vi "Limelight.vi"() -> (1 "RightTargetNorm":T1, 3 "LeftTargetNorm":T1)   [LabVIEW 2018]
uses:
  Util/Math/Vector/Vector3D.ctl
  5bda4818-5db7-4a37-94fe-e126cb2a47b4.vi
  65baa005-36a5-4b5c-ad00-e7831b38fc40.vi
  ffe1e7bf-722c-4abf-afb3-08bbb05ce56e.vi
  cfa8c977-f46c-4ebb-8e7e-f5b631340d2e.vi
  20f04a56-a653-4d81-a16d-e2cce2d6ced9.vi
  75f726a3-edf9-46da-8158-0b1851abcaf1.vi
  6606baff-e82b-4fed-8c44-0260f9793549.vi
  <vilib>/Array/Sort 2D Array - Pop Stack.vi
  <vilib>/Array/Sort 2D Array - Push Stack.vi
  <vilib>/Rock Robotics/Network Tables/NT Read Numeric Array.vi
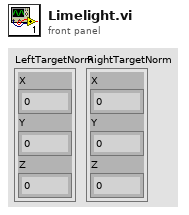
[diagram p1: front panel]
types:
  T1 = typedef "Vector3D.ctl" = cluster{"X":dbl, "Y":dbl, "Z":dbl}
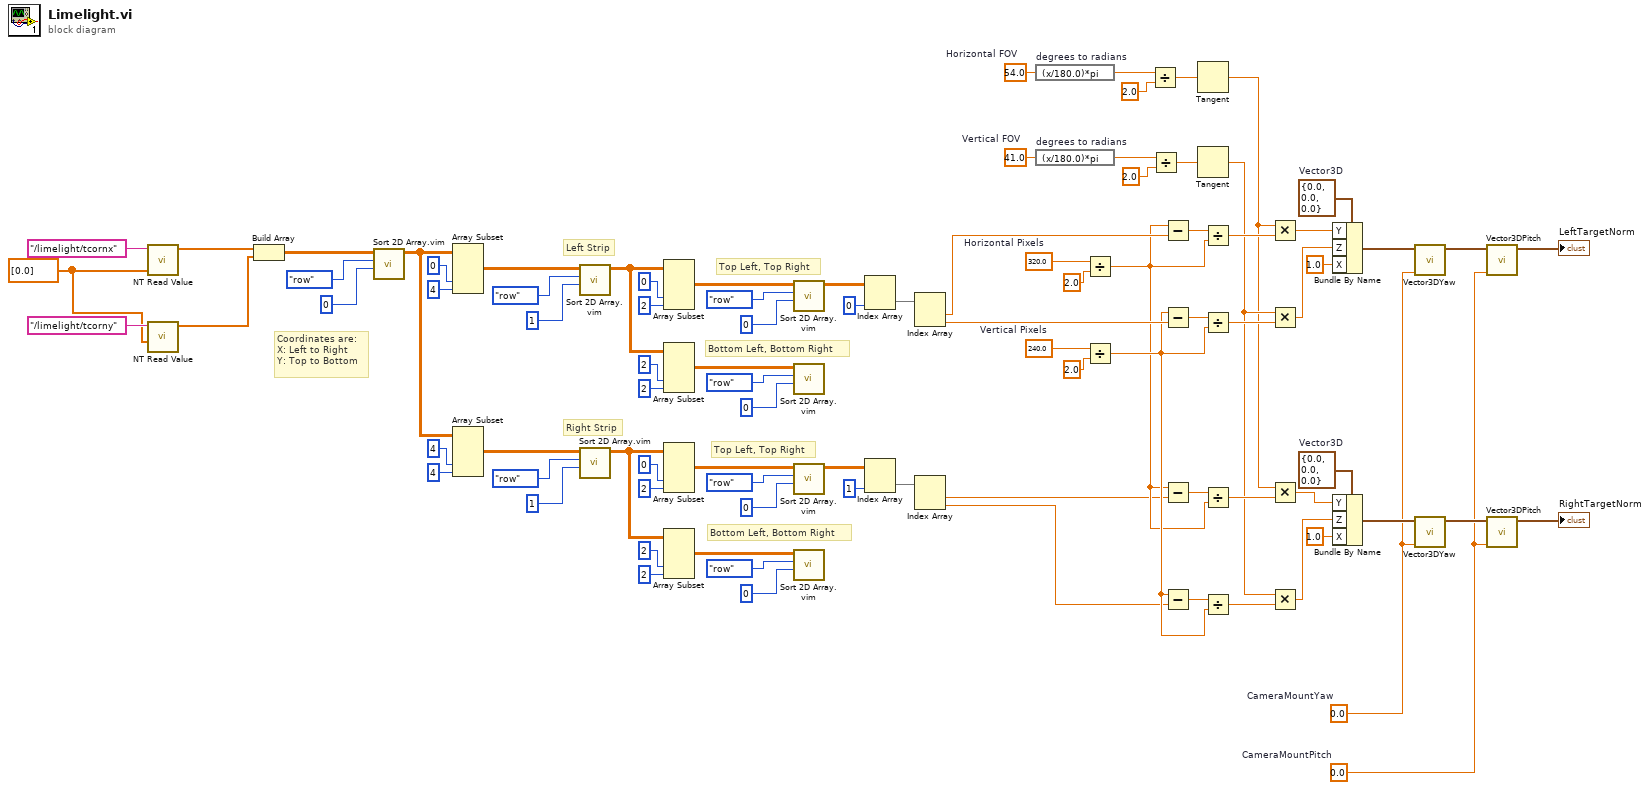
[diagram p0: block diagram]
diagram:
  w2 = 0.0  # CameraMountPitch
  w1 = 0.0  # CameraMountYaw
  w19 = T1 {"X"=0.0, "Y"=0.0, "Z"=0.0}  # Vector3D
  w32 = 320.0  # Horizontal Pixels
  w24 = T1 {"X"=0.0, "Y"=0.0, "Z"=0.0}  # Vector3D
  w38 = 240.0  # Vertical Pixels
  w41 = 54.0  # Horizontal FOV
  w44 = 41.0  # Vertical FOV
  w87 = dbl[] [0.0] ("Default Value")
  # "Coordinates are:\nX: Left to Right\nY: Top to Bottom"
  # "Top Left, Top Right"
  # "Bottom Left, Bottom Right"
  # "Top Left, Top Right"
  # "Bottom Left, Bottom Right"
  # "Right Strip"
  # "Left Strip"
  n1 = call-poly <vilib>:"NT Read Value.vi"("Default Value"=w87, "Name"="/limelight/tcornx") -> ("Numeric Array"=w89:dbl[])  [unwired: 8 in, 1 out]
  n2 = call-poly <vilib>:"NT Read Value.vi"("Default Value"=w87, "Name"="/limelight/tcorny") -> ("Numeric Array"=w88:dbl[])  [unwired: 8 in, 1 out]
  n3 = Build Array(w89, w88) -> (w84:dbl[][])
  n4 = call "Sort 2D Array.vim"("index"=0, "dimension to index (column)"=enum16{"column", "row"}."row", "2D array"=w84) -> ("sorted 2D array"=w79:dbl[][])  [unwired: 7 in, 1 out]
  n5 = Array Subset(array=w79, index (col)=0 ("index"), length (col)=4 ("index")) -> (w76:dbl[][])  [unwired: 2 in]
  n6 = Array Subset(array=w79, index (col)=4 ("index"), length (col)=4 ("index")) -> (w73:dbl[][])  [unwired: 2 in]
  n7 = call "Sort 2D Array.vim"("index"=1, "dimension to index (column)"=enum16{"column", "row"}."row", "2D array"=w76) -> ("sorted 2D array"=w68:dbl[][])  [unwired: 7 in, 1 out]
  n8 = call "Sort 2D Array.vim"("index"=1, "dimension to index (column)"=enum16{"column", "row"}."row", "2D array"=w73) -> ("sorted 2D array"=w63:dbl[][])  [unwired: 7 in, 1 out]
  n9 = Array Subset(array=w68, index (col)=0 ("index"), length (col)=2 ("index")) -> (w60:dbl[][])  [unwired: 2 in]
  n10 = Array Subset(array=w68, index (col)=2 ("index"), length (col)=2 ("index")) -> (w57:dbl[][])  [unwired: 2 in]
  n11 = Array Subset(array=w63, index (col)=0 ("index"), length (col)=2 ("index")) -> (w52:dbl[][])  [unwired: 2 in]
  n12 = Array Subset(array=w63, index (col)=2 ("index"), length (col)=2 ("index")) -> (w51:dbl[][])  [unwired: 2 in]
  n13 = call "Sort 2D Array.vim"("index"=0, "dimension to index (column)"=enum16{"column", "row"}."row", "2D array"=w60) -> ("sorted 2D array"=w48:dbl[][])  [unwired: 7 in, 1 out]
  n14 = call "Sort 2D Array.vim"("index"=0, "dimension to index (column)"=enum16{"column", "row"}."row", "2D array"=w57) -> ()  [unwired: 7 in, 2 out]
  n15 = call "Sort 2D Array.vim"("index"=0, "dimension to index (column)"=enum16{"column", "row"}."row", "2D array"=w52) -> ("sorted 2D array"=w47:dbl[][])  [unwired: 7 in, 1 out]
  n16 = call "Sort 2D Array.vim"("index"=0, "dimension to index (column)"=enum16{"column", "row"}."row", "2D array"=w51) -> ()  [unwired: 7 in, 2 out]
  n17 = Index Array(array=w48, index (col)=0 ("disabled index (col)")) -> (element=w46:dbl[])  [unwired: 1 in]
  n18 = Index Array(array=w47, index (col)=1 ("disabled index (col)")) -> (element=w45:dbl[])  [unwired: 1 in]
  n19 = Index Array(array=w46) -> (element #1=w5:dbl, element #2=w16:dbl)  [unwired: 2 in]
  n20 = Index Array(array=w45) -> (element #1=w3:dbl, element #2=w14:dbl)  [unwired: 2 in]
  n21 = expression code="(x/180.0)*pi" "degrees to radians"(w41) -> (w34:dbl)
  n22 = expression code="(x/180.0)*pi" "degrees to radians"(w44) -> (w42:dbl)
  n23 = Divide(x=w32, y=2.0) -> (x/y=w4:dbl)
  n24 = Divide(x=w38, y=2.0) -> (x/y=w15:dbl)
  n25 = Divide(x=w34, y=2.0) -> (x/y=w35:dbl)
  n26 = Divide(x=w42, y=2.0) -> (x/y=w40:dbl)
  n27 = Subtract(x=w4, y=w5) -> (x-y=w31:dbl)
  n28 = Subtract(x=w15, y=w16) -> (x-y=w39:dbl)
  n29 = Subtract(x=w4, y=w3) -> (x-y=w30:dbl)
  n30 = Subtract(x=w15, y=w14) -> (x-y=w29:dbl)
  n31 = Tangent(1:w35) -> (0:w9:dbl)
  n32 = Tangent(1:w40) -> (0:w10:dbl)
  n33 = Divide(x=w31, y=w4) -> (x/y=w28:dbl)
  n34 = Divide(x=w39, y=w15) -> (x/y=w25:dbl)
  n35 = Divide(x=w30, y=w4) -> (x/y=w27:dbl)
  n36 = Divide(x=w29, y=w15) -> (x/y=w26:dbl)
  n37 = Multiply(x=w9, y=w28) -> (x*y=w23:dbl)
  n38 = Multiply(x=w10, y=w25) -> (x*y=w22:dbl)
  n39 = Multiply(x=w9, y=w27) -> (x*y=w18:dbl)
  n40 = Multiply(x=w10, y=w26) -> (x*y=w17:dbl)
  n41 = Bundle By Name(cluster=w24, "Y"=w23, "Z"=w22, "X"=1.0 ("Z")) -> (w8:T1)
  n42 = Bundle By Name(cluster=w19, "Y"=w18, "Z"=w17, "X"=1.0 ("Z")) -> (w13:T1)
  n43 = call "Vector3DYaw.vi"("Vector3D"=w8, "Theta"=w1) -> ("Rotated Vector3D"=w6:T1)  [unwired: 8 in]
  n44 = call "Vector3DYaw.vi"("Vector3D"=w13, "Theta"=w1) -> ("Rotated Vector3D"=w12:T1)  [unwired: 8 in]
  n45 = call "Vector3DPitch.vi"("Vector3D"=w6, "Theta"=w2) -> ("Rotated Vector3D"=→"LeftTargetNorm":T1)  [unwired: 8 in]
  n46 = call "Vector3DPitch.vi"("Vector3D"=w12, "Theta"=w2) -> ("Rotated Vector3D"=→"RightTargetNorm":T1)  [unwired: 8 in]
